vi "Wait (boolean).vi"(8 "Time to wait (ms)":i32, 11 "In":bool) -> (3 "Out":bool)   [LabVIEW 2018]
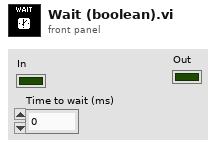
[diagram p1: front panel]
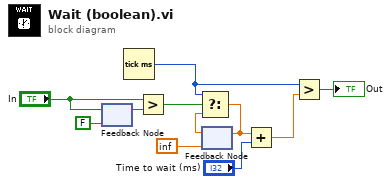
[diagram p0: block diagram]
diagram:
  n1 = feedback #1(FALSE ("Boolean")) -> (w10:bool)
  n2 = feedback-in #1("In") -> ()
  n3 = Tick Count (ms)() -> (millisecond timer value=w4:u32)
  n4 = Greater?(x="In", y=w10) -> (0:w8:bool)
  n5 = feedback #2(inf) -> (w7:dbl)
  n6 = Select(t=w4, s=w8, f=w7) -> (s? t:f=w6:dbl)
  n7 = feedback-in #2(w6) -> ()
  n8 = Add(x=w6, y="Time to wait (ms)") -> (x+y=w3:dbl)
  n9 = Greater?(x=w4, y=w3) -> (0:→"Out":bool)
